vi "visa2gpib.vi"(8 "error in":errorcluster, 11 "VISA in":refnum<visa-resource-name>) -> (0 "error out":errorcluster, 2 "combined address":string, 3 "VISA out":refnum<visa-resource-name>)   [LabVIEW 2020]
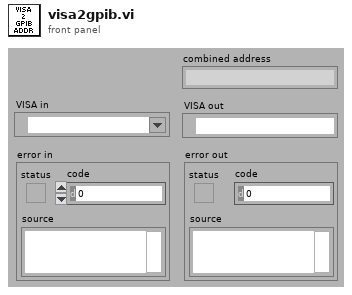
[diagram p1: front panel]
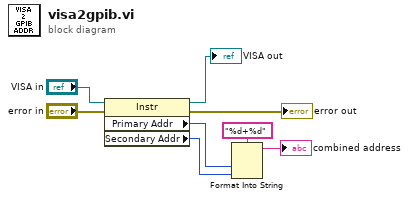
[diagram p0: block diagram]
diagram:
  n1 = property class="Instr"(reference="VISA in", error in="error in") -> (reference out=→"VISA out":refnum<visa-resource-name>, error out=→"error out":errorcluster, "Primary Addr"=w7:u16, "Secondary Addr"=w6:u16)
  n2 = Format Into String(format string="%d+%d", w7, w6) -> (resulting string=→"combined address":string)  [unwired: 2 in, 1 out]
